vi "launcher.vi"() -> ()   [LabVIEW 2019]
panel:
  out "Running":i32
  in  "stop":bool
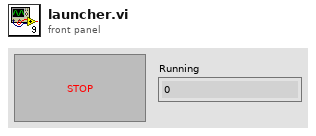
[diagram p1: front panel]
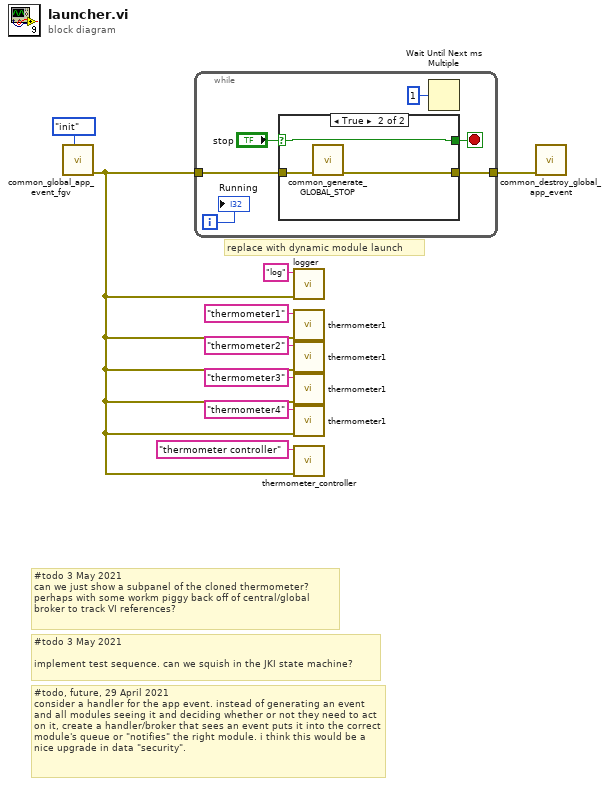
[diagram p0: block diagram]
diagram:
  # "#todo 3 May 2021\ncan we just show a subpanel of the cloned thermometer? perhaps with some workm piggy back off of central/global broker to track VI references?"
  # "#todo 3 May 2021\n\nimplement test sequence. can we squish in the JKI state machine?"
  # "#todo, future, 29 April 2021\nconsider a handler for the app event. instead of generating an event and all modules seeing it and deciding whether or not they need to act on it, create a handler/broker that sees an event puts it into the correct module's queue or \"notifies\" the right module. i think this would be a nice upgrade in data \"security\"."
  # "replace with dynamic module launch"
  n1 = call "common_global_app_event_fgv.vi"("action (0: get)"=enum16{"get", "init"}."init") -> ("error out"=w1:errorcluster)  [unwired: 9 in, 1 out]
  n2 = while {
    tunnel: w1 -> [w12]
    tunnel: [w11] -> w5
    i -> [w10]
    stop <- w14 stop-if-true
    n3 = case shown="True" "stop" {
      selector: "stop" -> [w17 w20]
      tunnel: [w17 w20] -> w14
      tunnel: w12 -> [w16 w18]
      tunnel: [w16 w19] -> w11
      frame False {
      }
      frame True {
        n4 = call "common_generate_GLOBAL_STOP.vi"("error in (no error)"=w18) -> ("error out"=w19:errorcluster)  [unwired: 10 in]
      }
    }
    n5 = Wait Until Next ms Multiple(millisecond multiple=u32 1 ("milliseconds to wait")) -> ()  [unwired: 1 out]
    "Running" <- w10
  }
  n6 = call "logger.vi"("error in (no error)"=w1, "module name"="log") -> ()  [unwired: 9 in, 1 out]
  n7 = call "thermometer1.vi"("error in (no error)"=w1, "module name"="thermometer1") -> ()  [unwired: 9 in, 1 out]
  n8 = call "thermometer1.vi"("error in (no error)"=w1, "module name"="thermometer2") -> ()  [unwired: 9 in, 1 out]
  n9 = call "thermometer1.vi"("error in (no error)"=w1, "module name"="thermometer3") -> ()  [unwired: 9 in, 1 out]
  n10 = call "thermometer1.vi"("error in (no error)"=w1, "module name"="thermometer4") -> ()  [unwired: 9 in, 1 out]
  n11 = call "thermometer_controller.vi"("error in (no error)"=w1, "module name"="thermometer controller") -> ()  [unwired: 9 in, 1 out]
  n12 = call "common_destroy_global_app_event.vi"("error in (no error)"=w5) -> ()  [unwired: 10 in, 1 out]
